vi "SaveAndPlayFile.vi"(8 "error in (no error)":errorcluster, 9 "Sound Format":T1={"sample rate (S/s)"=22050.0, "number of channels"=2, "bits per sample"=16}, 10 "Waveform(s) in":waveform(dbl)[](array[waveform]), 11 "Speaker device ID":u32 format="%.0x") -> (0 "error out":errorcluster)   [LabVIEW 2019]
uses:
  <vilib>/sound2/lvsound2.llb/Sound File Write (DBL).vi
  <vilib>/sound2/lvsound2.llb/Sound File Write Open.vi
  <vilib>/sound2/lvsound2.llb/Sound Data Format.ctl
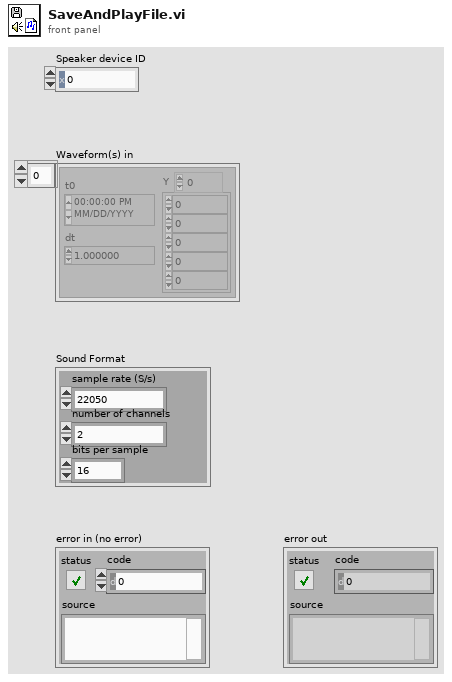
[diagram p1: front panel]
types:
  T1 = typedef "Sound Data Format.ctl" = cluster{"sample rate (S/s)":dbl, "number of channels":i32, "bits per sample":i32}
  T2 = typedef "Sound File Refnum.ctl" = refnum<file>
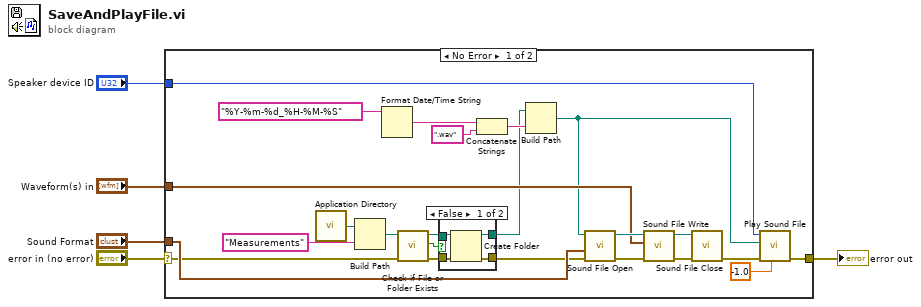
[diagram p0: block diagram]
diagram:
  n1 = case shown="No Error" "error in (no error)" {
    selector: "error in (no error)" -> [w16 w36]
    tunnel: [w9 w36] -> w5
    tunnel: "Waveform(s) in" -> [w18 _]
    tunnel: "Sound Format" -> [w17 _]
    tunnel: "Speaker device ID" -> [w7 _]
    frame No Error {
      n2 = call <vilib>:"Application Directory.vi"() -> ("Application Directory"=w19:path)
      n3 = Build Path(base path=w19, name or relative path="Measurements") -> (appended path=w12:path)
      n4 = Format Date/Time String(time format string (%c)="%Y-%m-%d_%H-%M-%S") -> (date/time string=w26:string)  [unwired: 2 in]
      n5 = call <vilib>:"Check if File or Folder Exists.vi"("error in (no error)"=w16, "path"=w12) -> ("error out"=w15:errorcluster, "file or folder exists?"=w11:bool, "dup path"=w13:path)  [unwired: 7 in]
      n6 = case shown="False" w11 {
        tunnel: w15 -> [w33 w34]
        tunnel: [w32 w34] -> w14
        tunnel: w13 -> [w31 w35]
        tunnel: [w30 w35] -> w10
        frame False {
          n7 = Create Folder(path (use dialog)=w31, error in=w33) -> (created path=w30:path, error out=w32:errorcluster)  [unwired: 1 in, 1 out]
        }
        frame True {
        }
      }
      n8 = Concatenate Strings(w26, ".wav" ("string")) -> (w28:string)
      n9 = Build Path(base path=w10, name or relative path=w28) -> (appended path=w8:path)
      n10 = call-poly <vilib>:"Sound File Open.vi"("error in (no error)"=w14, "sound format"=w17, "path"=w8) -> ("error out"=w24:errorcluster, "sound file refnum"=w25:T2)  [unwired: 7 in]
      n11 = call-poly <vilib>:"Sound File Write.vi"("error in (no error)"=w24, "data"=w18, "sound file refnum"=w25) -> ("error out"=w23:errorcluster, "sound file refnum out"=w22:T2)  [unwired: 7 in]
      n12 = call <vilib>:"Sound File Close.vi"("error in (no error)"=w23, "sound file refnum"=w22) -> ("error out"=w21:errorcluster)  [unwired: 9 in]
      n13 = call <vilib>:"Play Sound File.vi"("timeout (sec)"=-1.0, "error in (no error)"=w21, "path"=w8, "device ID"=w7) -> ("error out"=w9:errorcluster)  [unwired: 6 in, 1 out]
    }
    frame Error {
    }
  }
  "error out" <- w5
